vi "Translation Stages.vi"(8 "error in (no error)":errorcluster, 11 "Translation Stages in":refnum<class "Translation Stages.lvclass">) -> (0 "error out":errorcluster, 3 "Translation Stages out":refnum<class "Translation Stages.lvclass">)   [LabVIEW 2023, in "Translation Stages.lvclass"]
uses:
  Translation Stages.lvclass
  Global/GPIB Numbers.vi
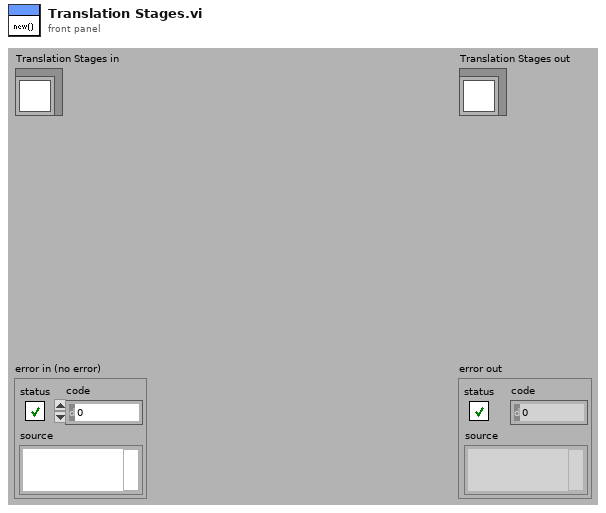
[diagram p1: front panel]
types:
  T1 = typedef "GPIB Type Def.ctl" = cluster{"Name":string, "bus":dbl, "GPIB":dbl, "GPIB as string":string, "byte":i32, "VISA Resource Name":refnum<visa-resource-name>}
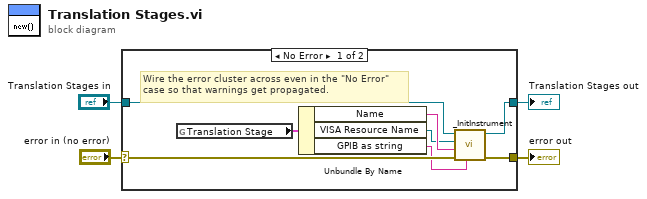
[diagram p0: block diagram]
diagram:
  n1 = case shown="No Error" "error in (no error)" {
    selector: "error in (no error)" -> [w10 w14]
    tunnel: [w9 w14] -> w3
    tunnel: [w11 w13] -> w1
    tunnel: "Translation Stages in" -> [w12 w13]
    frame No Error {
      # "Wire the error cluster across even in the \"No Error\"\ncase so that warnings get propagated."
      n2 = global read "GPIB Numbers.vi" "Translation Stage"() -> (w8:T1)
      n3 = Unbundle By Name(w8) -> ("Name"=w7:string, "VISA Resource Name"=w6:refnum<visa-resource-name>, "GPIB as string"=w5:string)
      n4 = call-dynamic "_InitInstrument.vi"("GPIB as string"=w5, "error in (no error)"=w10, "Name"=w7, "VISA Resource Name"=w6, "Instrument in"=w12) -> ("error out"=w9:errorcluster, "Instrument out"=w11:refnum<class "Translation Stages.lvclass">)  [unwired: 1 in, 4 out]
    }
    frame Error {
    }
  }
  "error out" <- w3
  "Translation Stages out" <- w1
